vi "Prueba.vi"() -> ()   [LabVIEW 2023]
uses:
  <vilib>/MakerHub/LINX/Public/Peripherals/Digital/Digital Read 1 Chan.vi
  <vilib>/MakerHub/LINX/Public/Peripherals/Digital/Digital Write 1 Chan.vi
  <vilib>/MakerHub/LINX/Public/Peripherals/Digital/Digital Read N Chans.vi
  <vilib>/MakerHub/LINX/Public/Peripherals/Digital/Digital Write N Chans.vi
  <vilib>/MakerHub/LINX/Private/Local IO/LinxDigitalRead.vi
  <vilib>/MakerHub/LINX/Public/Utilities/Check Channel.vi
  <vilib>/MakerHub/LINX/Private/Local IO/LinxDigitalWrite.vi
  <vilib>/MakerHub/LINX/Public/Utilities/Open Serial.vi
  <vilib>/MakerHub/LINX/Private/Utilties/Generate Error.vi
  <vilib>/MakerHub/LINX/LMH-LINX.lvlib
panel:
  out "Frecuencia":dbl
  in  "lectura":u8
  in  "Frecuencia (Hz)":u32(knob) scale=0.0..2000.0
  in  "Salida Digital":u8
  in  "stop":bool
  in  "Serial Port":refnum<visa-resource-name>="N/A"
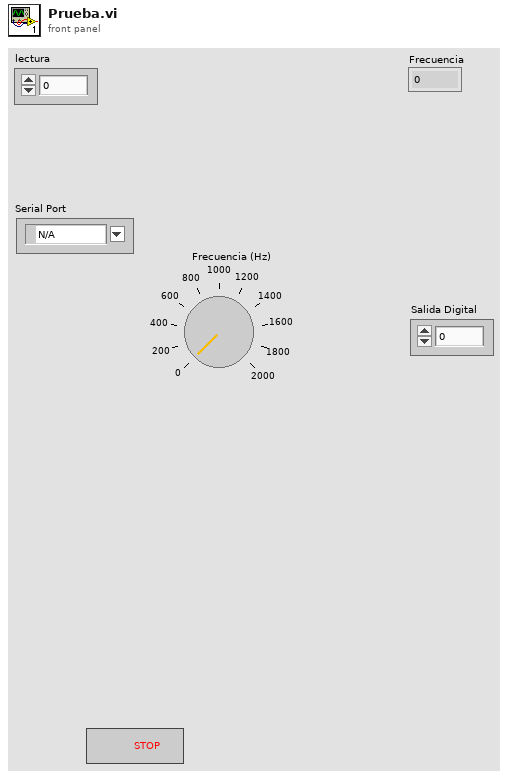
[diagram p1: front panel]
types:
  T1 = typedef "LMH-LINX.lvlib/LINX Ref.ctl" = cluster{"IO":T2, "Interface":T3, "LINX Device Config":T4}
  T2 = typedef "LMH-LINX.lvlib/Platform.ctl" = enum16{"Remote", "Local"}
  T3 = typedef "LMH-LINX.lvlib/Interface.ctl" = enum16{"Serial", "TCP"}
  T4 = typedef "LMH-LINX.lvlib/Device.lvlib/LINX Device Config.ctl" = cluster{"Interface":T3, "COM Port":refnum<visa-resource-name>, "TCP Configuration":T5, "Device Family":u8, "Device ID":u8, "Device Name":string, "TCP Ref":refnum<k5>, "Channels":T6}
  T5 = typedef "LMH-LINX.lvlib/Device.lvlib/TCP Config.ctl" = cluster{"IP Address":string, "Port":u16}
  T6 = typedef "LMH-LINX.lvlib/Channels.ctl" = cluster{"DI":u8[], "DO":u8[], "AI":u8[], "AO":u8[], "PWM":u8[], "QE":u8[], "UART":u8[], "I2C 2":u8[], "SPI":u8[], "CAN":u8[], "Servo":u8[], "AI Ref (V)":dbl, "AI Resolution (Bits)":u8, "AO Ref (V)":dbl, "AO Resolution (Bits)":u8}
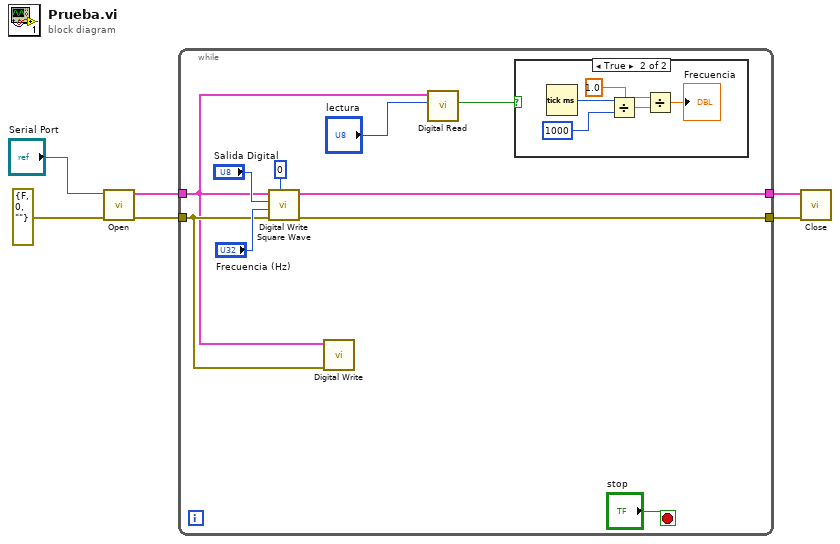
[diagram p0: block diagram]
diagram:
  n1 = call-poly <vilib>:"Open.vi"("Error In"=errorcluster {"status"=FALSE, "code"=0, "source"=""}, "Serial Port"="Serial Port") -> ("Error Out"=w6:errorcluster, "LINX Resource"=w5:T1)  [unwired: 7 in, 1 out]
  n2 = while {
    tunnel: w6 -> [w10]
    tunnel: w5 -> [w9]
    tunnel: [w14] -> w2
    tunnel: [w15] -> w1
    stop <- "stop" stop-if-true
    n3 = call <vilib>:"Digital Write Square Wave.vi"("Duration (ms)"=u32 0, "Error In"=w10, "Frequency (Hz)"="Frecuencia (Hz)", "Channel"="Salida Digital", "LINX Resource"=w9) -> ("Error Out"=w15:errorcluster, "LINX Resource"=w14:T1)  [unwired: 5 in]
    n4 = call-poly <vilib>:"Digital Write.vi"("Error In"=w10, "LINX Resource"=w9) -> ()  [unwired: 8 in, 2 out]
    n5 = call-poly <vilib>:"Digital Read.vi"("DI Channel"="lectura", "LINX Resource"=w9) -> ("DI Value"=w7:bool)  [unwired: 7 in, 2 out]
    n6 = case shown="True" w7 {
      frame False {
      }
      frame True {
        n7 = Tick Count (ms)() -> (millisecond timer value=w21:u32)
        n8 = Divide(x=w21, y=u32 1000) -> (x/y=w19:dbl)
        n9 = Divide(x=1.0, y=w19) -> (x/y=→"Frecuencia":dbl)
      }
    }
  }
  n10 = call <vilib>:"Close.vi"("Error In"=w1, "LINX Resource"=w2) -> ()  [unwired: 9 in, 1 out]
